vi "Configure Voltage Setpoint.vi"(0 "reference in":refnum<class "BKP-911x Power Supply.lvclass">, 2 "Voltage Setpoint (V)":dbl format="%.3g", 5 "error in (no error)":errorcluster) -> (14 "reference out":refnum<class "BKP-911x Power Supply.lvclass">, 19 "error out":errorcluster)   [LabVIEW 2020, in "BKP-911x Power Supply.lvclass"]
uses:
  BKP-911x Power Supply.lvclass
  <instrlib>/BK Precision 911X Series/BK Precision 911X Series.lvlib
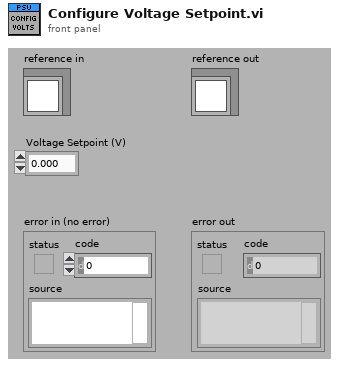
[diagram p1: front panel]
types:
  T1 = typedef "BKP-911x Power Supply.lvclass/ObjectAttributes.ctl" = cluster{"VISA resource name":refnum<visa-resource-name>, "Simulated?":bool, "Latest Values":dbl[], "Signal List":T2[], "Voltage Setpoint (V)":dbl, "Current Limit (A)":dbl, "Output Enabled?":bool}
  T2 = typedef "IO Signal List.ctl" = enum16{"Timestamp", "PSU_FB_U_VDC", "PSU_FB_I_AMP", "PSU_FB_W_WATT", "PSU_CMD_U_VDC", "PSU_CMD_I_AMP", "PSU_CMD_OUTPUT", "LCR_PRIMARY", "LCR_SECONDARY", "UV_R_Ohm", "UW_R_Ohm", "VW_R_Ohm", "UV_L_H", "UW_L_H", "VW_L_H", "U_U_VDC", "V_U_VDC", "W_U_VDC", "U_I_AMP", "V_I_AMP", "W_I_AMP", "PWM_CMD_DC_%", "PWM_CMD_VDC", "PWM_CMD_Hz", "PWM_FB_DC_%", "PWM_FB_VDC", "PWM_FB_Hz", "DO_RELAY_U_LCR_A", "DO_RELAY_V_LCR_A", "DO_RELAY_V_LCR_B", "DO_RELAY_W_LCR_B", "DIFF_UV_UW_L_H", "DIFF_UV_VW_L_H", "DIFF_UW_VW_L_H", "DIFF_UV_UW_R_Ohm", "DIFF_UV_VW_R_Ohm", "DIFF_UW_VW_R_Ohm", "DIFF_UV_U_VDC", "DIFF_UW_U_VDC", "DIFF_VW_U_VDC"}
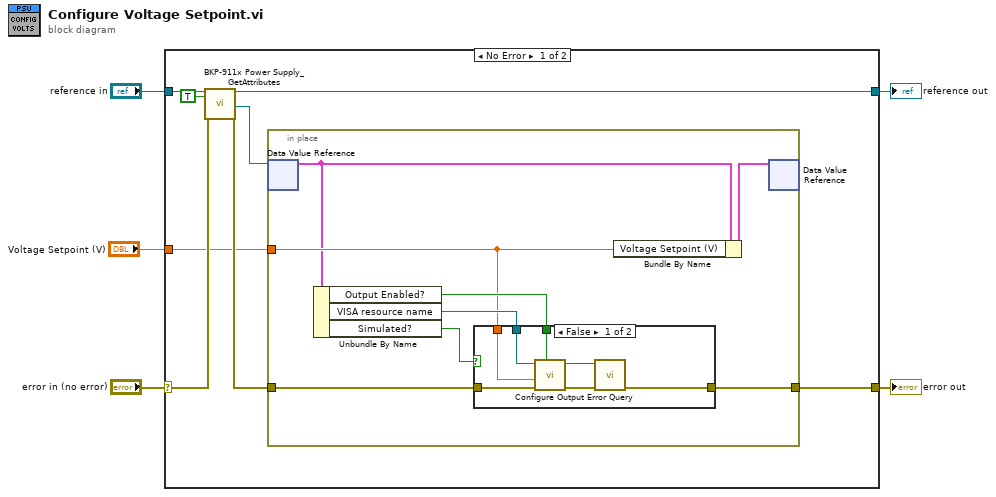
[diagram p0: block diagram]
diagram:
  n1 = case shown="No Error" "error in (no error)" {
    selector: "error in (no error)" -> [w13 w31]
    tunnel: [w9 w31] -> w4
    tunnel: [w11 w30] -> w2
    tunnel: "reference in" -> [w12 w30]
    tunnel: "Voltage Setpoint (V)" -> [w8 _]
    frame No Error {
      n2 = call "BKP-911x Power Supply_GetAttributes.vi"("reference in"=w12, "OnlyGetDvrReference(False)"=TRUE, "error in (no error)"=w13) -> ("reference out"=w11:refnum<class "BKP-911x Power Supply.lvclass">, "DataRef"=w7:refnum<data-value>, "error out"=w10:errorcluster)  [unwired: 13 in, 1 out]
      n3 = in-place {
        in-place-border: w10 -> [w21]
        in-place-border: [w20] -> w9
        in-place-border: w8 -> [w17]
        n4 = in-place-dvr #1(w7) -> (w15:T1)  [unwired: 1 out]
        n5 = Unbundle By Name(w15) -> ("Output Enabled?"=w19:bool, "VISA resource name"=w18:refnum<visa-resource-name>, "Simulated?"=w16:bool)
        n6 = case shown="False" w16 {
          tunnel: w21 -> [w28 w29]
          tunnel: [w22 w29] -> w20
          tunnel: w19 -> [w27 _]
          tunnel: w18 -> [w26 _]
          tunnel: w17 -> [w25 _]
          frame False {
            n7 = call <instrlib>:"Configure Output.vi"("Enable Output (T: Enable)"=w27, "error in (no error)"=w28, "Voltage Level (0.0 V)"=w25, "VISA resource name"=w26) -> ("error out"=w24:errorcluster, "VISA resource name out"=w23:refnum<visa-resource-name>)  [unwired: 6 in]
            n8 = call <instrlib>:"Error Query.vi"("error in (no error)"=w24, "VISA resource name"=w23) -> ("error out"=w22:errorcluster)  [unwired: 6 in, 3 out]
          }
          frame True {
          }
        }
        n9 = Bundle By Name(cluster=w15, "Voltage Setpoint (V)"=w17) -> (w14:T1)
        n10 = in-place-dvr #1(w14) -> ()  [unwired: 2 out]
      }
    }
    frame Error {
    }
  }
  "error out" <- w4
  "reference out" <- w2
